vi "_allan_open_file.vi"(8 "保存ファイル名":string, 9 "ファイルパス名":path=path "c:/Data") -> (0 "ファイルopen-error":errorcluster, 1 "refnum data":refnum<file>, 2 "refnum allan":refnum<file>, 3 "refnum_fft":refnum<file>, 4 "refnum temp":refnum<file>)   [LabVIEW 2017]
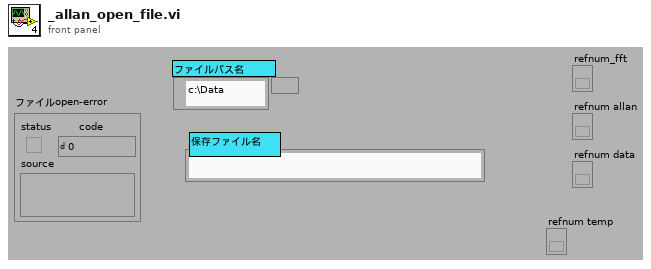
[diagram p1: front panel]
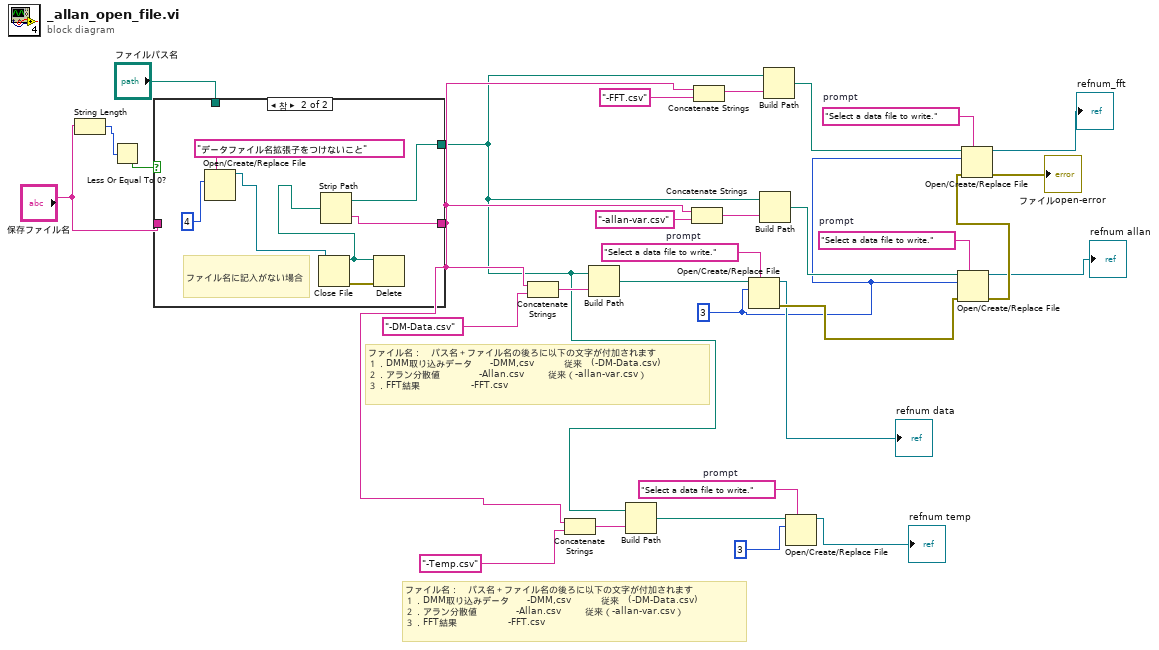
[diagram p0: block diagram]
diagram:
  w2 = "Select a data file to write."  # prompt
  w9 = 3
  w23 = "Select a data file to write."  # prompt
  w29 = "Select a data file to write."  # prompt
  w31 = "Select a data file to write."  # prompt
  # "ファイル名：　パス名＋ファイル名の後ろに以下の文字が付加されます\n１．DMM取り込みデータ　　-DMM,csv    　　従来　(-DM-Data.csv)\n２．アラン分散値             -Allan.csv        従来（-allan-var.csv）\n３．FFT結果                 -FFT.csv"
  # "ファイル名：　パス名＋ファイル名の後ろに以下の文字が付加されます\n１．DMM取り込みデータ　　-DMM,csv    　　従来　(-DM-Data.csv)\n２．アラン分散値             -Allan.csv        従来（-allan-var.csv）\n３．FFT結果                 -FFT.csv"
  n1 = String Length(string="保存ファイル名") -> (length=w16:i32)
  n2 = Less Or Equal To 0?(x=w16) -> (x <= 0?=w15:bool)
  n3 = case shown="참" w15 {
    tunnel: [w33 w38] -> w4
    tunnel: "保存ファイル名" -> [w33 _]
    tunnel: [w32 w39] -> w3
    tunnel: "ファイルパス名" -> [w32 _]
    frame False {
      # "ファイル名記入ありの場合"
    }
    frame True {
      # "ファイル名に記入がない場合"
      n4 = Open/Create/Replace File(prompt="データファイル名拡張子をつけないこと", operation (0:open)=4) -> (refnum out=w37:refnum<file>)  [unwired: 4 in, 2 out]
      n5 = Close File(refnum=w37) -> (path=w34:path, error out=w35:errorcluster)  [unwired: 1 in]
      n6 = Strip Path(path=w34) -> (stripped path=w39:path, name=w38:string)
      n7 = Delete(path (use dialog)=w34, error in=w35) -> ()  [unwired: 3 in, 3 out]
    }
  }
  n8 = Concatenate Strings(w4, "-DM-Data.csv") -> (w27:string)
  n9 = Concatenate Strings(w4, "-Temp.csv") -> (w7:string)
  n10 = Build Path(base path=w3, name or relative path=w27) -> (appended path=w26:path)
  n11 = Build Path(base path=w3, name or relative path=w7) -> (appended path=w6:path)
  n12 = Concatenate Strings(w4, "-allan-var.csv") -> (w25:string)
  n13 = Concatenate Strings(w4, "-FFT.csv") -> (w20:string)
  n14 = Open/Create/Replace File(file path (use dialog)=w26, prompt=w31, operation (0:open)=w9) -> (refnum out=→"refnum data":refnum<file>, error out=w19:errorcluster)  [unwired: 3 in, 1 out]
  n15 = Build Path(base path=w3, name or relative path=w25) -> (appended path=w24:path)
  n16 = Build Path(base path=w3, name or relative path=w20) -> (appended path=w22:path)
  n17 = Open/Create/Replace File(file path (use dialog)=w6, prompt=w2, operation (0:open)=3) -> (refnum out=→"refnum temp":refnum<file>)  [unwired: 3 in, 2 out]
  n18 = Open/Create/Replace File(file path (use dialog)=w24, error in=w19, prompt=w29, operation (0:open)=w9) -> (refnum out=→"refnum allan":refnum<file>, error out=w18:errorcluster)  [unwired: 2 in, 1 out]
  n19 = Open/Create/Replace File(file path (use dialog)=w22, error in=w18, prompt=w23, operation (0:open)=w9) -> (refnum out=→"refnum_fft":refnum<file>, error out=→"ファイルopen-error":errorcluster)  [unwired: 2 in, 1 out]
